vi "getValidPacketRange.vi"(11 "MQTTVersion50 in":refnum<class "MQTTVersion50.lvclass">) -> (1 "Lower Range":u8=1 format="%02x", 2 "Upper Range":u8=14 format="%02x", 3 "MQTTVersion50 out":refnum<class "MQTTVersion50.lvclass">)   [LabVIEW 2013, in "MQTT_Control_Packets_50.lvlib" / "MQTTVersion50.lvclass"]
uses:
  MQTTVersion50.lvclass
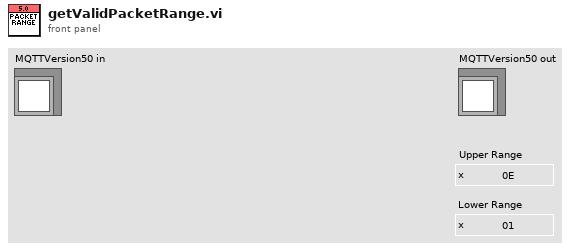
[diagram p1: front panel]
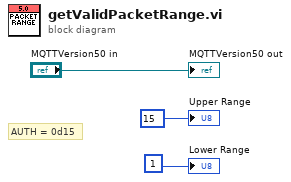
[diagram p0: block diagram]
diagram:
  # "AUTH = 0d15"
  "MQTTVersion50 out" <- "MQTTVersion50 in"
  "Upper Range" <- u8 15 ("Byte")
  "Lower Range" <- u8 1 ("Byte")
